vi "HQ Main.vi"() -> ()   [LabVIEW 2017]
uses:
  Type Defs/PodHealth.ctl
  Type Defs/PodStates.ctl
  Type Defs/PodState.ctl
panel:
  out "Pod States":T1
  out "Pusher Attached":bool
  in  "Phase":T2={"Pre-Flight Tests"=FALSE, "Ready"=FALSE, "Accelerate"=TRUE, "Coast"=FALSE, "Brake"=FALSE, "Post-Flight"=FALSE}
  in  "Detail Window":T3(tab)
  in  "Reset Sensors":bool
  in  "Vent":bool
  in  "Brake Boost":bool
  in  "Brake Open":bool
  in  "Sensor Power":bool
  in  "Activate Pneumatics":bool
  in  "Friction Brake":bool
  in  "Mag Brake":bool
  in  "Levitation":bool
  in  "Reset Laser Count":bool
  out "Acceleration (m/s^2)":dbl(graph)
  out "Velocity (m/s)":dbl(graph)
  out "Position":T4(graph)
  out "Pressure":T4(graph)
  out "Levitation Gap (mm)":T5(graph)
  out "Battery Monitor":cluster{"Voltage (Total)":dbl, "Power":dbl}(graph)={"Voltage (Total)"=11.91201, "Power"=9.516504789}
  in  "Run ToF Calibration":bool=TRUE
  in  "Send Non-Critical Data":bool=TRUE
  in  "Stop":bool
  out "Battery Current":dbl(knob)=9.144776890538314 scale=0.0..5.0
  out "Battery Voltage":dbl(knob)=11.942438656676648 scale=11.0..12.0
  out "Batt. Temp":dbl(slide)=81.63265306122449 scale=0.0..100.0
  out "Gap 4":u8(slide)=11 scale=0.0..100.0
  out "Gap 3":u8(slide)=10 scale=0.0..200.0
  out "Gap 2":u8(slide)=12 scale=0.0..100.0
  out "Gap 1":u8(slide)=13 scale=0.0..100.0
  out "Track Position":dbl(slide)=438.0053908355795 scale=0.0..5000.0
  out "Pod Health":T6={"Overall Pod Health"=TRUE, "Power"={"Power"=TRUE, "Friction Brakes"=TRUE, "Magnetic Brakes"=TRUE, "Primary Battery"=TRUE, "Backup Battery"=TRUE}, "Pressure"={"Pressure"=TRUE, "HP"=TRUE, "MP "=TRUE, "LP"=TRUE}, "Position"={"Position"=TRUE, "Maglock"=TRUE, "Levitation (ToF)"=TRUE}}
  # "TBD kick off calibration on ToF"
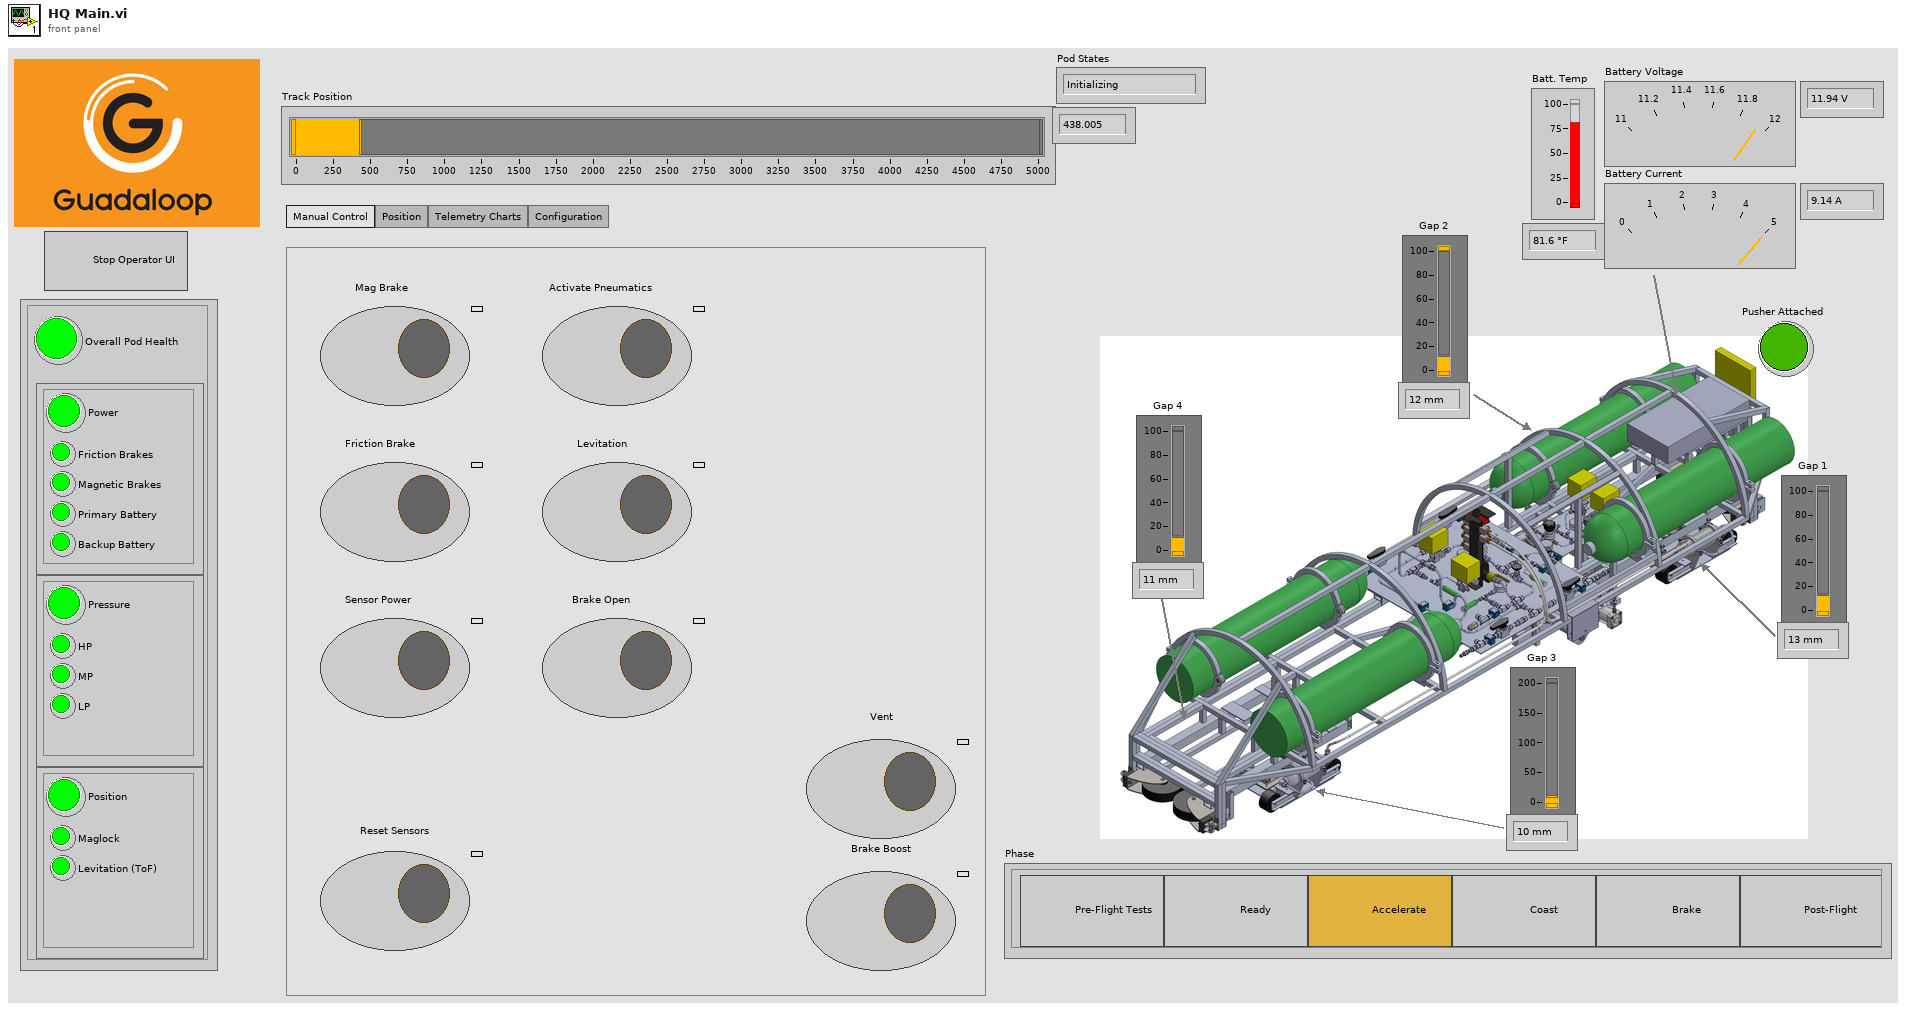
[diagram p1: front panel]
types:
  T1 = typedef "PodState.ctl" = enum16{"Initializing", "Pre-flight Testing", "Ready", "Pushing", "Coast", "Braking", "Post-flight", "Fault"}
  T2 = typedef "PodStates.ctl" = cluster{"Pre-Flight Tests":bool, "Ready":bool, "Accelerate":bool, "Coast":bool, "Brake":bool, "Post-Flight":bool}
  T3 = enum32{"Manual Control", "Position", "Telemetry Charts", "Configuration"}
  T4 = cluster{"Double":dbl, "Double":dbl, "Double":dbl, "Double":dbl}
  T5 = cluster{"UInt8":u8, "UInt8":u8, "UInt8":u8, "UInt8":u8}
  T6 = typedef "PodHealth.ctl" = cluster{"Overall Pod Health":bool, "Power":cluster{"Power":bool, "Friction Brakes":bool, "Magnetic Brakes":bool, "Primary Battery":bool, "Backup Battery":bool}, "Pressure":cluster{"Pressure":bool, "HP":bool, "MP ":bool, "LP":bool}, "Position":cluster{"Position":bool, "Maglock":bool, "Levitation (ToF)":bool}}
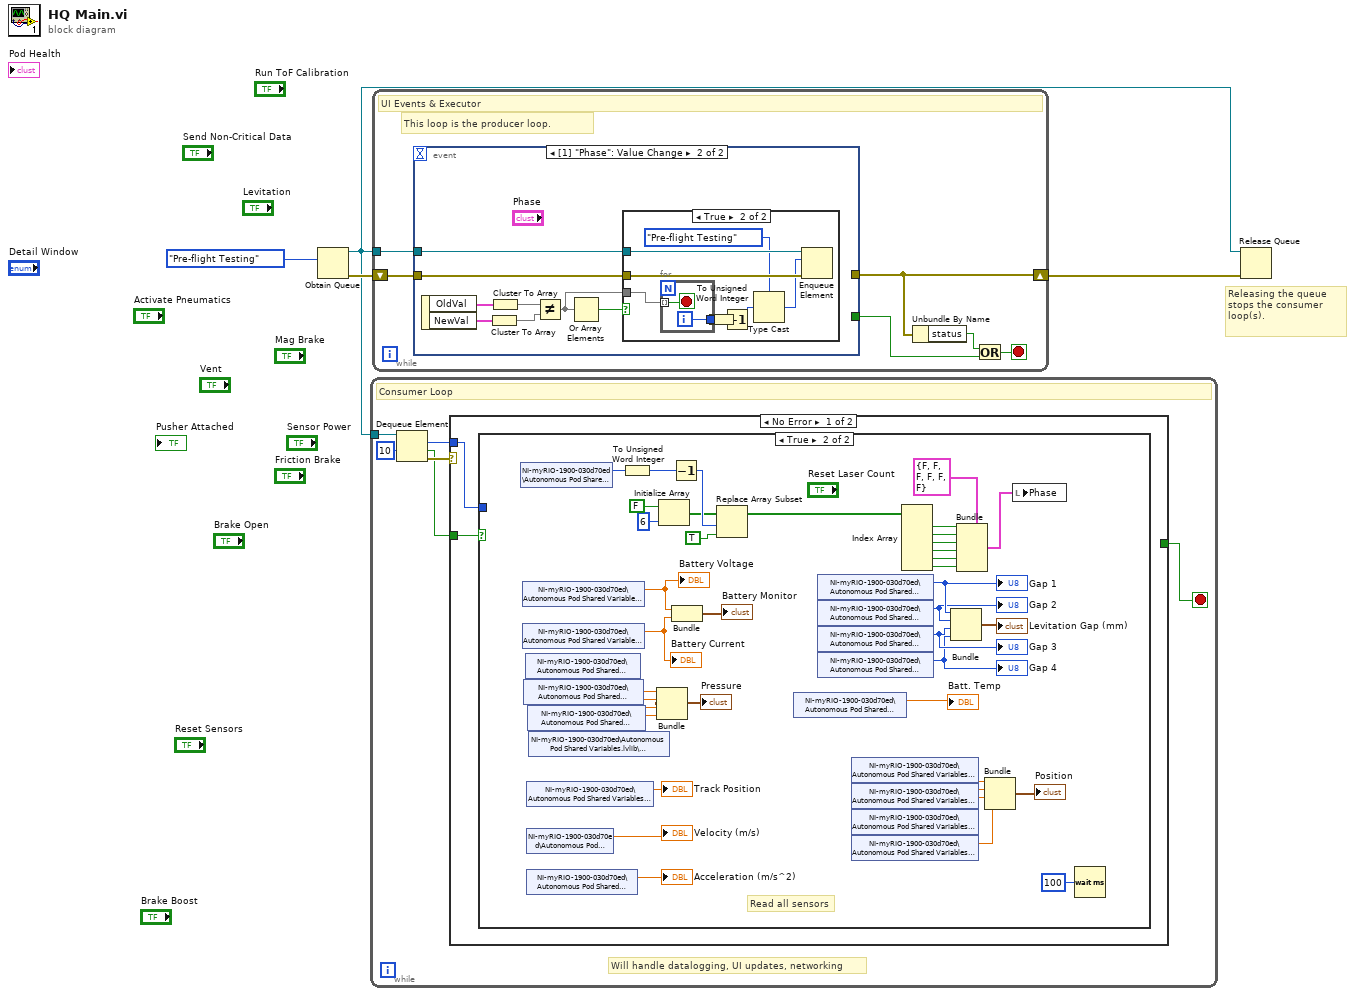
[diagram p0: block diagram]
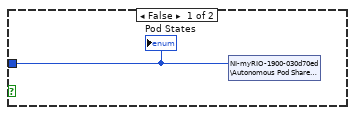
[diagram p2: hidden frame]
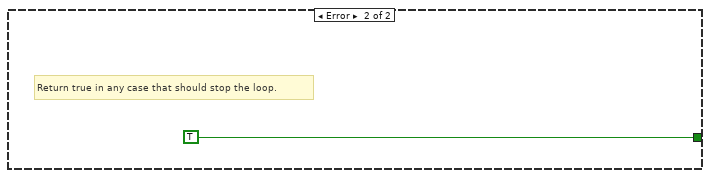
[diagram p3: hidden frame]
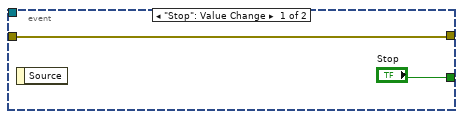
[diagram p4: hidden frame]
diagram:
  # "Releasing the queue stops the consumer loop(s)."
  n1 = Obtain Queue(element data type=PodState."Pre-flight Testing" ("Pod States")) -> (queue out=w2:refnum<queue>, error out=w4:errorcluster)  [unwired: 4 in, 1 out]
  n2 = while {
    tunnel: w2 -> [w10]
    stop <- w7 stop-if-true
    # "Will handle datalogging, UI updates, networking"
    # "Consumer Loop"
    n3 = Dequeue Element(queue=w10, timeout in ms (-1)=10) -> (element=w8:T1, timed out?=w5:bool, error out=w9:errorcluster)  [unwired: 1 in, 1 out]
    n4 = case shown="No Error" w9 {
      tunnel: w8 -> [w11 _]
      tunnel: [_ TRUE] -> w7
      tunnel: w5 -> [w12 _]
      frame No Error {
        n5 = case shown="True" w12 {
          tunnel: w11 -> [w13 _]
          frame False {
            n6 = shared-variable "NI-myRIO-1900-030d70ed\\Autonomous Pod Shared Variables.lvlib\\PodState"(w13) -> ()  [unwired: 1 in, 1 out]
            "Pod States" <- w13
          }
          frame True {
            # "Read all sensors"
            n7 = shared-variable "NI-myRIO-1900-030d70ed\\Autonomous Pod Shared Variables.lvlib\\PodState"() -> (w52:T1)  [unwired: 1 in, 1 out]
            n8 = shared-variable "NI-myRIO-1900-030d70ed\\Autonomous Pod Shared Variables.lvlib\\BatteryVoltage"() -> (w28:dbl)  [unwired: 1 in, 1 out]
            "Battery Voltage" <- w28
            n9 = shared-variable "NI-myRIO-1900-030d70ed\\Autonomous Pod Shared Variables.lvlib\\BatteryCurrent"() -> (w27:dbl)  [unwired: 1 in, 1 out]
            "Battery Current" <- w27
            n10 = shared-variable "NI-myRIO-1900-030d70ed\\Autonomous Pod Shared Variables.lvlib\\UtilityPressure"() -> (w34:dbl)  [unwired: 1 in, 1 out]
            n11 = shared-variable "NI-myRIO-1900-030d70ed\\Autonomous Pod Shared Variables.lvlib\\HighPressure"() -> (w35:dbl)  [unwired: 1 in, 1 out]
            n12 = shared-variable "NI-myRIO-1900-030d70ed\\Autonomous Pod Shared Variables.lvlib\\PositionSLaser2"() -> (→"Track Position":dbl)  [unwired: 1 in, 1 out]
            n13 = shared-variable "NI-myRIO-1900-030d70ed\\Autonomous Pod Shared Variables.lvlib\\Velocity"() -> (→"Velocity (m/s)":dbl)  [unwired: 1 in, 1 out]
            n14 = shared-variable "NI-myRIO-1900-030d70ed\\Autonomous Pod Shared Variables.lvlib\\Acceleration"() -> (→"Acceleration (m/s^2)":dbl)  [unwired: 1 in, 1 out]
            n15 = shared-variable "NI-myRIO-1900-030d70ed\\Autonomous Pod Shared Variables.lvlib\\BrakePressure"() -> (w33:dbl)  [unwired: 1 in, 1 out]
            n16 = shared-variable "NI-myRIO-1900-030d70ed\\Autonomous Pod Shared Variables.lvlib\\LevitationPressure"() -> (w32:dbl)  [unwired: 1 in, 1 out]
            n17 = To Unsigned Word Integer(number=w52) -> (unsigned 16bit integer=w38:u16)
            n18 = Bundle("Double"=w35, "Double"=w34, "Double"=w33, "Double"=w32) -> (→"Pressure":T4)  [unwired: 1 in]
            n19 = Initialize Array(FALSE, 6 ("dimension size")) -> (w41:bool[])
            n20 = Decrement(x=w38) -> (x-1=w43:u16)
            n21 = Bundle("Double"=w28, "Double"=w27) -> (→"Battery Monitor":cluster{"Double":dbl, "Double":dbl})  [unwired: 1 in]
            n22 = Replace Array Subset(array=w41, new element=TRUE, index=w43) -> (w45:bool[])
            n23 = shared-variable "NI-myRIO-1900-030d70ed\\Autonomous Pod Shared Variables.lvlib\\BatteryTemp"() -> (→"Batt. Temp":dbl)  [unwired: 1 in, 1 out]
            n24 = shared-variable "NI-myRIO-1900-030d70ed\\Autonomous Pod Shared Variables.lvlib\\ToF1Distance"() -> (w26:u8)  [unwired: 1 in, 1 out]
            "Gap 1" <- w26
            n25 = shared-variable "NI-myRIO-1900-030d70ed\\Autonomous Pod Shared Variables.lvlib\\ToF2Distance"() -> (w25:u8)  [unwired: 1 in, 1 out]
            "Gap 2" <- w25
            n26 = shared-variable "NI-myRIO-1900-030d70ed\\Autonomous Pod Shared Variables.lvlib\\ToF3Distance"() -> (w24:u8)  [unwired: 1 in, 1 out]
            "Gap 3" <- w24
            n27 = shared-variable "NI-myRIO-1900-030d70ed\\Autonomous Pod Shared Variables.lvlib\\ToF4Distance"() -> (w23:u8)  [unwired: 1 in, 1 out]
            "Gap 4" <- w23
            n28 = shared-variable "NI-myRIO-1900-030d70ed\\Autonomous Pod Shared Variables.lvlib\\PositionFLaser1"() -> (w20:dbl)  [unwired: 1 in, 1 out]
            n29 = shared-variable "NI-myRIO-1900-030d70ed\\Autonomous Pod Shared Variables.lvlib\\PositionFLaser2"() -> (w19:dbl)  [unwired: 1 in, 1 out]
            n30 = shared-variable "NI-myRIO-1900-030d70ed\\Autonomous Pod Shared Variables.lvlib\\PositionSLaser1"() -> (w18:dbl)  [unwired: 1 in, 1 out]
            n31 = shared-variable "NI-myRIO-1900-030d70ed\\Autonomous Pod Shared Variables.lvlib\\PositionSLaser2"() -> (w17:dbl)  [unwired: 1 in, 1 out]
            n32 = Index Array(array=w45) -> (element #1=w46:bool, element #2=w47:bool, element #3=w48:bool, element #4=w49:bool, element #5=w50:bool, element #6=w51:bool)  [unwired: 6 in]
            n33 = Bundle("UInt8"=w26, "UInt8"=w25, "UInt8"=w24, "UInt8"=w23) -> (→"Levitation Gap (mm)":T5)  [unwired: 1 in]
            n34 = Bundle(cluster=T2 {"Pre-Flight Tests"=FALSE, "Ready"=FALSE, "Accelerate"=FALSE, "Coast"=FALSE, "Brake"=FALSE, "Post-Flight"=FALSE} ("Phase"), "Pre-Flight Tests"=w46, "Ready"=w47, "Accelerate"=w48, "Coast"=w49, "Brake"=w50, "Post-Flight"=w51) -> (w37:T2)
            n35 = Bundle("Double"=w20, "Double"=w19, "Double"=w18, "Double"=w17) -> (→"Position":T4)  [unwired: 1 in]
            n36 = local write "Phase"(w37) -> ()
            n37 = Wait (ms)(milliseconds to wait=u32 100) -> ()  [unwired: 1 out]
          }
        }
      }
      frame Error {
        # "Return true in any case that should stop the loop."
      }
    }
  }
  n38 = while {
    shift-right: [w55] -> w3
    shift-left: w4 -> [w58]
    tunnel: w2 -> [w59]
    stop <- w56 stop-if-true
    # "This loop is the producer loop."
    # "UI Events & Executor"
    n39 = event shown="[1] \"Phase\": Value Change" {
      selector: _ -> [_ _]
      dyn-events: _ -> [_ _]
      timeout: _ -> [_ _]
      tunnel: w59 -> [_ w68]
      tunnel: w58 -> [w61 w67]
      tunnel: [w61 _] -> w55
      tunnel: ["Stop" _] -> w57
      event "Stop": Value Change {
        n40 = event-data() -> ()  [unwired: 1 in, 1 out]
      }
      event Value Change {
        n41 = event-data() -> ("OldVal"=w69:T2, "NewVal"=w66:T2)  [unwired: 1 in]
        n42 = Cluster To Array(cluster=w66) -> (array=w64:bool[])
        n43 = Cluster To Array(cluster=w69) -> (array=w65:bool[])
        n44 = Not Equal?(x=w65, y=w64) -> (x != y?=w62:bool[])
        n45 = Or Array Elements(Boolean array=w62) -> (logical OR=w63:bool)
        n46 = case shown="True" w63 {
          tunnel: w68 -> [_ w77]
          tunnel: w67 -> [_ w76]
          tunnel: w62 -> [_ w75]
          frame False {
          }
          frame True {
            n47 = for {
              tunnel: w75 -> [w79] mode=indexing
              tunnel: [w78] -> w74
              i -> [w78]
              stop <- w79 stop-if-true
            }
            n48 = To Unsigned Word Integer(number=w74) -> (unsigned 16bit integer=w70:u16)
            n49 = Increment(x=w70) -> (x+1=w71:u16)
            n50 = Type Cast(type=PodState."Pre-flight Testing" ("Pod States"), x=w71) -> (*(type *) &x=w72:T1)
            n51 = Enqueue Element(queue=w77, element=w72, error in (no error)=w76) -> ()  [unwired: 1 in, 3 out]
          }
        }
      }
    }
    n52 = Unbundle By Name(w55) -> ("status"=w54:bool)
    n53 = Or(x=w54, y=w57) -> (x .or. y?=w56:bool)
  }
  n54 = Release Queue(queue=w2, error in (no error)=w3) -> ()  [unwired: 1 in, 3 out]
